vi "Update Internal State.vi"(8 "error in (no error)":errorcluster, 11 "Routing and Faulting Item Ref in":T1 format="%.0x") -> (0 "error out":errorcluster, 3 "Routing and Faulting Item Ref out":T1 format="%.0x")   [LabVIEW 2017, in "Routing and Faulting System Explorer.lvlib"]
uses:
  Routing and Faulting System Explorer.lvlib
  <vilib>/NI Veristand/Custom Device API/Custom Device Item Ref.ctl
  <vilib>/NI Veristand/Custom Device Tools/Custom Device Utility Library/Search Direction.ctl
  Shared/Constants.vi
  <vilib>/NI Veristand/Custom Device Tools/Custom Device Utility Library/NI VeriStand - Search for Item by GUID.vi
  Scripting/Routing and Faulting Scripting.lvlib
  <vilib>/NI Veristand/Custom Device Tools/Custom Device Utility Library/Custom Device Utility Library.lvlib
  Shared/Routing and Faulting Shared.lvlib
  <vilib>/NI Veristand/Custom Device API/Custom Device API.lvlib
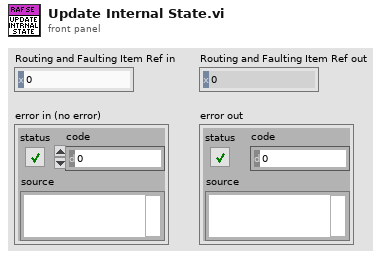
[diagram p1: front panel]
types:
  T1 = typedef "Custom Device API.lvlib/Custom Device Item Ref.ctl" = u64
  T2 = typedef "Custom Device Utility Library.lvlib/Search Direction.ctl" = enum16{"Down", "Up"}
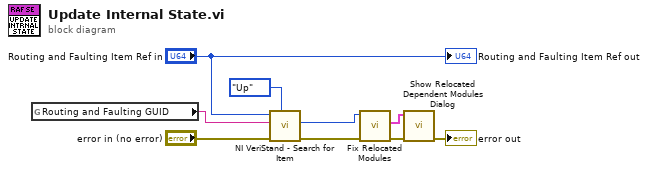
[diagram p0: block diagram]
diagram:
  n1 = global read "Constants.vi" "Routing and Faulting GUID"() -> (w2:string)
  n2 = call-poly <vilib>:"NI VeriStand - Search for Item.vi"("Direction (Down)"=Search_Direction."Up", "error in"="error in (no error)", "Item GUID"=w2, "Section Ref in"="Routing and Faulting Item Ref in") -> ("error out"=w4:errorcluster, "Item Ref"=w1:T1)  [unwired: 4 in, 2 out]
  n3 = call "Fix Relocated Modules.vi"("error in (no error)"=w4, "Routing and Faulting Ref in"=w1) -> ("error out"=w8:errorcluster, "Relocated Dependent Modules"=w7:cluster{"Old Path":string, "New Path":string}[])  [unwired: 6 in, 2 out]
  n4 = call "Show Relocated Dependent Modules Dialog.vi"("error in (no error)"=w8, "Relocated Dependent Modules"=w7) -> ("error out"=→"error out":errorcluster)  [unwired: 9 in]
  "Routing and Faulting Item Ref out" <- "Routing and Faulting Item Ref in"
